vi "dinner menu sub vi.vi"() -> ()   [LabVIEW 2019]
panel:
  out "SPECIALTY SALADS":string
  out "VEGETABLES":string
  out "CARVED MEATS & POULTRY":string
  out "POTATO & RICE ACCOMPANIMENTS":string
  out "DINNER ENTREES":string
  out "Desert":string
  out "before substring":string
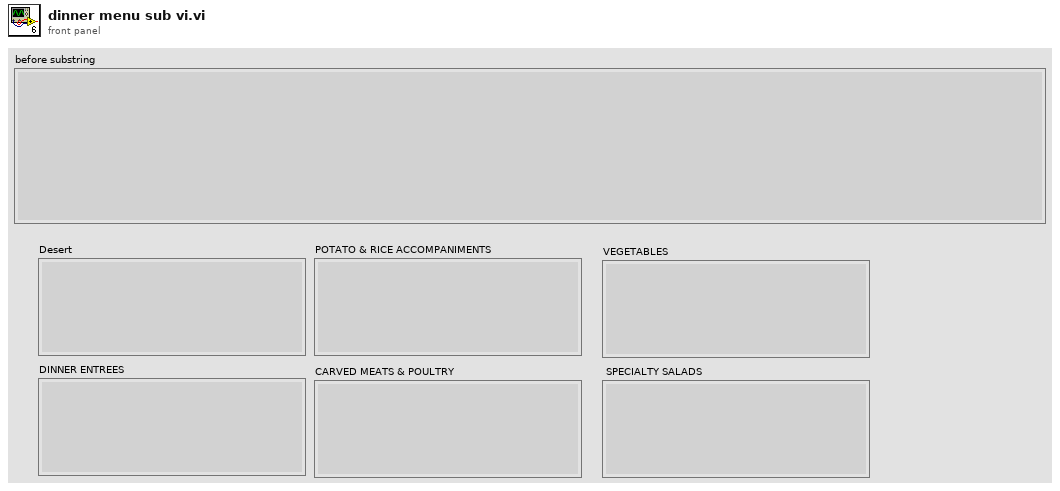
[diagram p1: front panel]
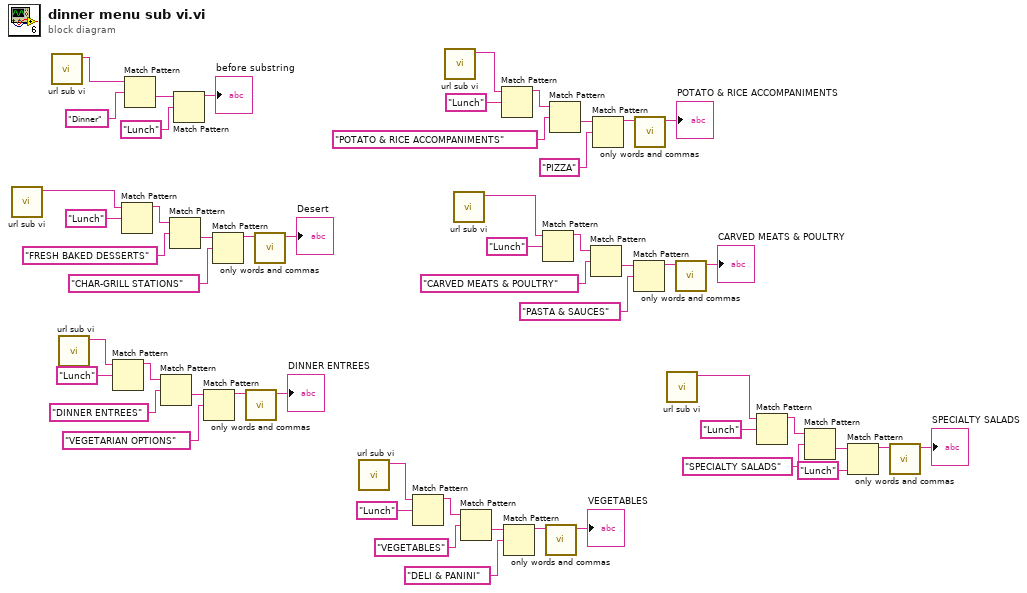
[diagram p0: block diagram]
diagram:
  n1 = call "url sub vi.vi"() -> ("body 2"=w6:string)  [unwired: 11 in]
  n2 = call "url sub vi.vi"() -> ("body 2"=w7:string)  [unwired: 11 in]
  n3 = call "url sub vi.vi"() -> ("body 2"=w5:string)  [unwired: 11 in]
  n4 = Match Pattern(string=w5, regular expression="Lunch") -> (before substring=w36:string)  [unwired: 1 in, 3 out]
  n5 = Match Pattern(string=w6, regular expression="Lunch") -> (before substring=w43:string)  [unwired: 1 in, 3 out]
  n6 = Match Pattern(string=w7, regular expression="Dinner") -> (after substring=w52:string)  [unwired: 1 in, 3 out]
  n7 = Match Pattern(string=w36, regular expression="DINNER ENTREES") -> (after substring=w41:string)  [unwired: 1 in, 3 out]
  n8 = Match Pattern(string=w43, regular expression="FRESH BAKED DESSERTS") -> (after substring=w48:string)  [unwired: 1 in, 3 out]
  n9 = Match Pattern(string=w52, regular expression="Lunch") -> (before substring=→"before substring":string)  [unwired: 1 in, 3 out]
  n10 = Match Pattern(string=w41, regular expression="VEGETARIAN OPTIONS") -> (before substring=w40:string)  [unwired: 1 in, 3 out]
  n11 = Match Pattern(string=w48, regular expression="CHAR-GRILL STATIONS") -> (before substring=w47:string)  [unwired: 1 in, 3 out]
  n12 = call "only words and commas.vi"("input string"=w40) -> ("result string"=→"DINNER ENTREES":string)  [unwired: 10 in]
  n13 = call "only words and commas.vi"("input string"=w47) -> ("result string"=→"Desert":string)  [unwired: 10 in]
  n14 = call "url sub vi.vi"() -> ("body 2"=w4:string)  [unwired: 11 in]
  n15 = Match Pattern(string=w4, regular expression="Lunch") -> (before substring=w16:string)  [unwired: 1 in, 3 out]
  n16 = call "url sub vi.vi"() -> ("body 2"=w1:string)  [unwired: 11 in]
  n17 = call "url sub vi.vi"() -> ("body 2"=w2:string)  [unwired: 11 in]
  n18 = Match Pattern(string=w16, regular expression="VEGETABLES") -> (after substring=w20:string)  [unwired: 1 in, 3 out]
  n19 = Match Pattern(string=w1, regular expression="Lunch") -> (before substring=w30:string)  [unwired: 1 in, 3 out]
  n20 = Match Pattern(string=w20, regular expression="DELI & PANINI") -> (before substring=w19:string)  [unwired: 1 in, 3 out]
  n21 = Match Pattern(string=w2, regular expression="Lunch") -> (before substring=w23:string)  [unwired: 1 in, 3 out]
  n22 = call "only words and commas.vi"("input string"=w19) -> ("result string"=→"VEGETABLES":string)  [unwired: 10 in]
  n23 = Match Pattern(string=w30, regular expression="POTATO & RICE ACCOMPANIMENTS") -> (after substring=w34:string)  [unwired: 1 in, 3 out]
  n24 = Match Pattern(string=w23, regular expression="CARVED MEATS & POULTRY") -> (after substring=w27:string)  [unwired: 1 in, 3 out]
  n25 = Match Pattern(string=w34, regular expression="PIZZA") -> (before substring=w33:string)  [unwired: 1 in, 3 out]
  n26 = Match Pattern(string=w27, regular expression="PASTA & SAUCES") -> (before substring=w26:string)  [unwired: 1 in, 3 out]
  n27 = call "only words and commas.vi"("input string"=w33) -> ("result string"=→"POTATO & RICE ACCOMPANIMENTS":string)  [unwired: 10 in]
  n28 = call "url sub vi.vi"() -> ("body 2"=w3:string)  [unwired: 11 in]
  n29 = call "only words and commas.vi"("input string"=w26) -> ("result string"=→"CARVED MEATS & POULTRY":string)  [unwired: 10 in]
  n30 = Match Pattern(string=w3, regular expression="Lunch") -> (before substring=w10:string)  [unwired: 1 in, 3 out]
  n31 = Match Pattern(string=w10, regular expression="SPECIALTY SALADS") -> (after substring=w14:string)  [unwired: 1 in, 3 out]
  n32 = Match Pattern(string=w14, regular expression="Lunch") -> (before substring=w13:string)  [unwired: 1 in, 3 out]
  n33 = call "only words and commas.vi"("input string"=w13) -> ("result string"=→"SPECIALTY SALADS":string)  [unwired: 10 in]
